vi "ex_Launch Express VI Help.vi"(4 "error in (no error)":errorcluster, 6 "Help File Path":path=path "<helpdir>/lvexpress.chm", 7 "Keyword/HTML File":string) -> (0 "error out":errorcluster)   [LabVIEW 2020]
doc: "Opens the online help file to the location specified by the Search Help String and Help File Path inputs."
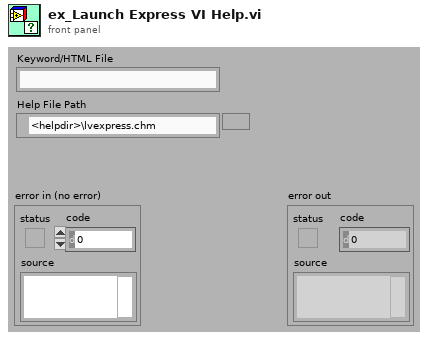
[diagram p1: front panel]
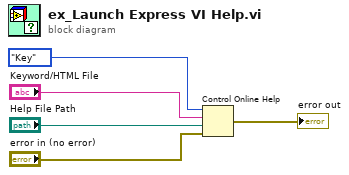
[diagram p0: block diagram]
diagram:
  n1 = Control Online Help(1:"error in (no error)", 2:"Help File Path", 3:"Keyword/HTML File", 4:enum16{"Contents", "Key", "Close"}."Key" ("Operation")) -> (0:→"error out":errorcluster)
